vi "SV TDMS Write Spectrum (Colormap).vi"(0 "tdms file":refnum<k34>, 5 "group name in":string="Colormap", 9 "colormap":T7, 11 "error in":errorcluster, 13 "spectrum info":T1 {"x-axis units" items=["Time (s)"=0, "Frequency-CB (Hz)"=1, "Frequency-CPB (Hz)"=1248, "Frequency-Arbitrary (Hz)"=2357, "Quefrency (s)"=2, "Revolutions (rev)"=3, "Order"=4, "Speed (RPM)"=11, "Speed (rad/s)"=21, "Index"=65535]; "weighting filter" items=["Linear", "A-weighting", "B-weighting", "C-weighting", "ITU-R 468-4", "Dolby", "CCITT", "C-message", "Wb", "Wc", "Wd", "We", "Wf", "Wh", "Wj", "Wk", "Wm", "AES17 20 kHz lowpass", "AES17 40 kHz lowpass", "AES17 20 kHz highpass", "AES17 40 kHz highpass"]; "dB reference [EU]" format="%.2f"; "engineering units" items=["custom..."=0, "V"=1, "A"=21, "C"=30, "pC"=31, "s"=32, "-"=29, "Pa"=2, "N"=20, "g"=3, "m/s^2"=4, "m/s"=5, "m"=6, "mm/s"=12, "mm"=13, "micron/s"=14, "micron"=15, "in/s^2"=7, "in/s"=8, "in"=9, "mil/s"=10, "mil"=11, "rad/s^2"=16, "rad/s"=17, "rad"=18, "deg/s^2"=26, "deg/s"=27, "deg"=28, "RPM"=22, "cycle/s^2"=23, "Hz"=24, "cycle"=25, "strain"=19]; "spectral info"."window" items=["None "=0, "Hanning"=1, "Hamming"=2, "Blackman-Harris"=3, "Exact Blackman"=4, "Blackman"=5, "Flat Top"=6, "4 Term B-Harris "=7, "7 Term B-Harris"=8, "Low Sidelobe"=9, "Force - Exponential"=10, "Gaussian"=62]}) -> (4 "tdms file out":refnum<k34>, 6 "group name out":string="Colormap", 15 "error out":errorcluster)   [LabVIEW 2017]
doc: "Writes data to the specified .tdms file in a format specific to the polymorphic instance. Wire data to the <B>scaled signal [EU]</B> input to determine the polymorphic instance to use or manually select the instance."
uses:
  <vilib>/addons/_NISVFA/_Shared subVIs/Controls/svc_Spectrum Info.ctl
  <vilib>/addons/_NISVFA/_Shared subVIs/Controls/svc_X-Axis Units.ctl
  <vilib>/addons/_NISVFA/_Shared subVIs/Controls/svc_Spectrum Type.ctl
  <vilib>/addons/_NISVFA/_Shared subVIs/Controls/svc_Engineering Units Text Ring.ctl
  <vilib>/addons/_NISVFA/_Shared subVIs/Controls/svc_Weighting Filter Text Ring.ctl
  <vilib>/addons/_NISVFA/_Shared subVIs/Controls/svc_Complimentary Spectrum Units.ctl
  <vilib>/addons/_NISVFA/_Shared subVIs/Controls/svc_Speed Profile.ctl
  <vilib>/addons/_NISVFA/_Shared subVIs/Controls/NI Channel Properties.ctl
  <vilib>/addons/_NISVFA/_Shared subVIs/Controls/LV Datatypes.ctl
  <vilib>/addons/_NISVFA/_Shared subVIs/Controls/NI Spectrum Component.ctl
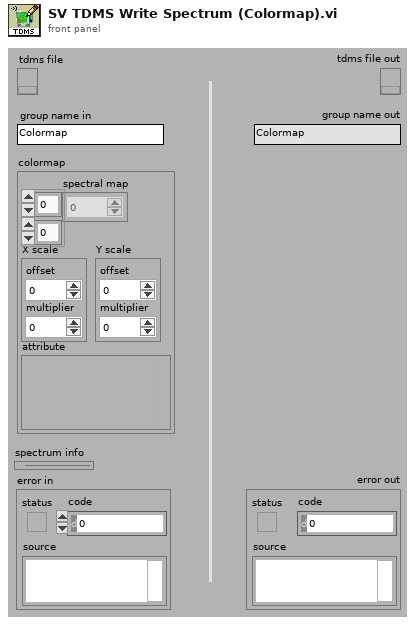
[diagram p1: front panel]
types:
  T1 = typedef "svc_Spectrum Info.ctl" = cluster{"channel name":string, "description":string, "x-axis units":T2, "spectral info":cluster{"spectrum type":T3, "linear/dB":enum16{"linear", "dB"}, "window":u16, "window size":i32, "FFT size":i32}, "engineering units":T4, "custom label":string, "dB reference [EU]":dbl, "peak units":enum16{"rms", "peak", "peak-peak"}, "weighting filter":T5, "spectral density?":bool, "unit label":string, "spectrum skewed?":bool, "complimentary spectrum units":T6}
  T2 = typedef "svc_X-Axis Units.ctl" = u16
  T3 = typedef "svc_Spectrum Type.ctl" = enum16{"FFT Spectrum [complex]", "Amplitude [Magnitude]", "Power [Magnitude^2]", "Cross Spectrum [complex]", "Frequency Response [Complex]"}
  T4 = typedef "svc_Engineering Units Text Ring.ctl" = u16
  T5 = typedef "svc_Weighting Filter Text Ring.ctl" = u16
  T6 = typedef "svc_Complimentary Spectrum Units.ctl" = enum16{"none", "radians", "degrees", "cycles", "imaginary"}
  T7 = cluster{"spectral map":dbl[][], "X scale":cluster{"offset":dbl, "multiplier":dbl}, "Y scale":cluster{"offset":dbl, "multiplier":dbl}, "attribute":variant}
  T8 = typedef "LV Datatypes.ctl" = i32
  T9 = typedef "NI Spectrum Component.ctl" = u16
  T10 = typedef "NI Channel Properties.ctl" = u16
  T11 = enum16{"Frequency-Time", "Time-Frequency", "Order-Time", "Time-Order", "Frequency-RPM", "RPM-Frequency", "Order-RPM", "RPM-Order"}
  T12 = typedef "svc_Speed Profile.ctl" = cluster{"time [s]":dbl[], "speed [RPM]":dbl[]}
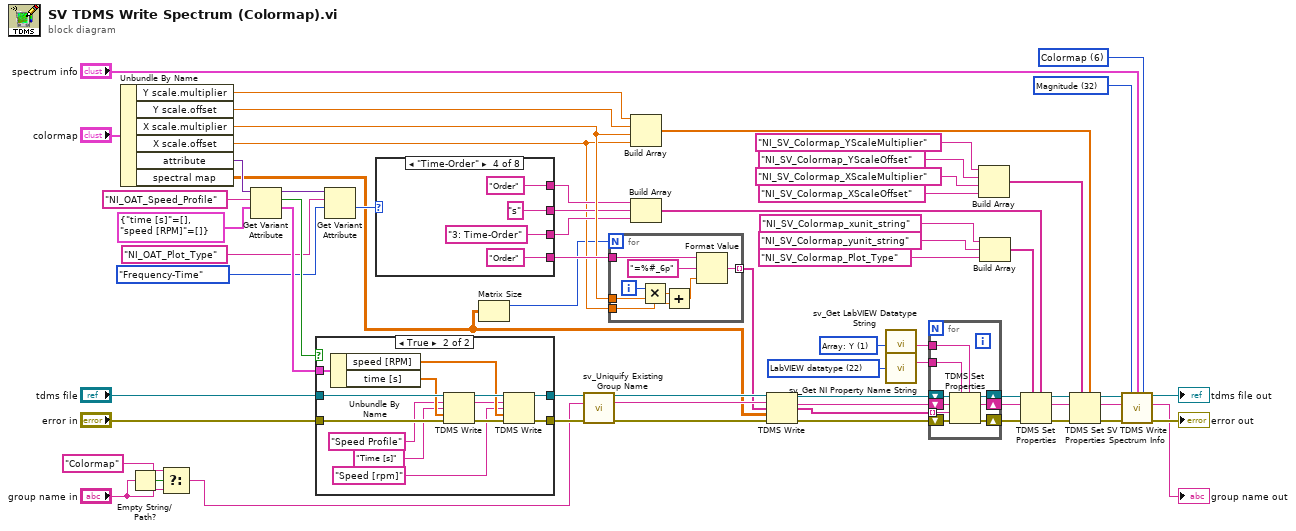
[diagram p0: block diagram]
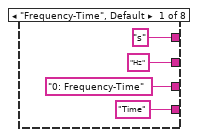
[diagram p2: hidden frame]
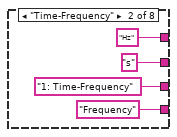
[diagram p3: hidden frame]
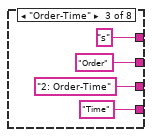
[diagram p4: hidden frame]
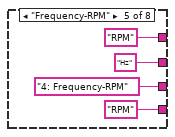
[diagram p5: hidden frame]
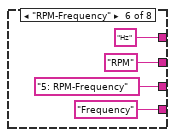
[diagram p6: hidden frame]
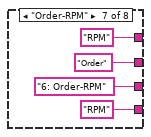
[diagram p7: hidden frame]
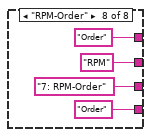
[diagram p8: hidden frame]
diagram:
  w35 = T8 6 items=["String: abc"=7, "Boolean: True or False"=8, "Scalar: y"=0, "Array: Y"=1, "Waveform: t0, dt, Y, variant"=2, "Cluster: x0, dx, Y"=3, "Cluster: X, Y"=4, "Waterfall"=5, "Colormap"=6] ("LabVIEW datatype")
  w41 = T9 32 items=["Magnitude"=32, "Phase"=33, "Real"=34, "Imaginary"=35, "Coherence"=36, "Unknown"=99] ("spectrum component")
  w52 = T8 1 items=["String: abc"=-2, "Boolean: True or False"=-1, "Scalar: y"=0, "Array: Y"=1, "Waveform: t0, dt, Y, variant"=2, "Cluster: x0, dx, Y"=3, "Cluster: X, Y"=4, "Waterfall"=5, "Colormap"=6] ("LabVIEW datatype")
  w53 = T10 22 items=["Channel name", "Channel description", "Y-axis label", "Y-axis unit string", "X-axis label", "X-axis unit string", "x0", "dx", "Number of samples", "X channel", "Filter settled", "dB reference", "Window", "Window parameter", "Window size", "FFT size", "Peak units", "Spectrum type", "Magnitude scale", "Spectral density", "Sensor sensitivity (mV/EU)", "X-axis domain", "LabVIEW datatype"] ("property")
  n1 = Unbundle By Name("colormap") -> ("Y scale.multiplier"=w28:dbl, "Y scale.offset"=w27:dbl, "X scale.multiplier"=w26:dbl, "X scale.offset"=w4:dbl, "attribute"=w60:variant, "spectral map"=w2:dbl[][])
  n2 = Empty String/Path?(string/path="group name in") -> (empty?=w64:bool)
  n3 = Select(t="Colormap" ("group name"), s=w64, f="group name in") -> (s? t:f=w3:string)
  n4 = Get Variant Attribute(Variant=w60, name="NI_OAT_Speed_Profile", default value (empty Variant)=T12 {"time [s]"=[], "speed [RPM]"=[]} ("speed profile")) -> (duplicate Variant=w61:variant, found=w59:bool, value=w58:T12)  [unwired: 1 in, 1 out]
  n5 = case shown="True" w59 {
    tunnel: "tdms file" -> [w68 w81]
    tunnel: "error in" -> [w67 w80]
    tunnel: [w67 w77] -> w38
    tunnel: [w68 w76] -> w40
    tunnel: w58 -> [_ w75]
    frame False {
    }
    frame True {
      n6 = Unbundle By Name(w75) -> ("speed [RPM]"=w73:dbl[], "time [s]"=w74:dbl[])
      n7 = TDMS Write(0:w81, 5:"Speed Profile" ("name"), 7:"Time [s]" ("name"), 9:w74, 11:w80) -> (4:w79:refnum<k34>, 6:w69:string, 15:w78:errorcluster)  [unwired: 1 in, 1 out]
      n8 = TDMS Write(0:w79, 5:w69, 7:"Speed [rpm]" ("name"), 9:w73, 11:w78) -> (4:w76:refnum<k34>, 15:w77:errorcluster)  [unwired: 1 in, 2 out]
    }
  }
  n9 = Get Variant Attribute(Variant=w61, name="NI_OAT_Plot_Type", default value (empty Variant)=T11."Frequency-Time" ("plot type")) -> (value=w31:T11)  [unwired: 1 in, 3 out]
  n10 = case shown="\"Time-Order\"" w31 {
    tunnel: ["s" ("name") "Hz" ("name") "s" ("name") "Order" ("name") "RPM" ("name") "Hz" ("name") "RPM" ("name") "Order" ("name")] -> w16
    tunnel: ["Hz" ("name") "s" ("name") "Order" ("name") "s" ("name") "Hz" ("name") "RPM" ("name") "Order" ("name") "RPM" ("name")] -> w15
    tunnel: ["0: Frequency-Time" "1: Time-Frequency" "2: Order-Time" "3: Time-Order" "4: Frequency-RPM" "5: RPM-Frequency" "6: Order-RPM" "7: RPM-Order"] -> w14
    tunnel: ["Time" ("name") "Frequency" ("name") "Time" ("name") "Order" ("name") "RPM" ("name") "Frequency" ("name") "RPM" ("name") "Order" ("name")] -> w30
    frame "Frequency-Time", Default {
    }
    frame "Time-Frequency" {
    }
    frame "Order-Time" {
    }
    frame "Time-Order" {
    }
    frame "Frequency-RPM" {
    }
    frame "RPM-Frequency" {
    }
    frame "Order-RPM" {
    }
    frame "RPM-Order" {
    }
  }
  n11 = Matrix Size(0:w2) -> (1:w1:i32)  [unwired: 1 out]
  n12 = call <vilib>:"sv_Uniquify Existing Group Name.vi"("tdms file ref"=w40, "group name"=w3, "error in"=w38) -> ("tdms file out"=w39:refnum<k34>, "unique group"=w36:string, "error out"=w37:errorcluster)  [unwired: 10 in]
  n13 = for {
    N: w1 -> [_]
    tunnel: [w121] -> w5 mode=indexing
    tunnel: w26 -> [w120]
    tunnel: w4 -> [w119]
    tunnel: w30 -> [w117]
    i -> [w118]
    n14 = Multiply(x=w118, y=w120) -> (x*y=w116:dbl)
    n15 = Add(x=w116, y=w119) -> (x+y=w115:dbl)
    n16 = Format Value(string ("")=w117, format string="=%#_6p", value (0)=w115) -> (output string=w121:string)
  }
  n17 = Build Array(w28, w27, w26, w4) -> (w17:dbl[])
  n18 = Build Array(w16, w15, w14) -> (w9:string[])
  n19 = TDMS Write(0:w39, 5:w36, 7:w5, 9:w2, 11:w37) -> (4:w49:refnum<k34>, 6:w50:string, 8:w48:string[], 15:w51:errorcluster)  [unwired: 1 in]
  n20 = call <vilib>:"sv_Get LabVIEW Datatype String.vi"("LabVIEW datatype"=w52) -> ("datatype string"=w47:string)  [unwired: 4 in]
  n21 = call <vilib>:"sv_Get NI Property Name String.vi"("property"=w53) -> ("TDMS property name"=w46:string)  [unwired: 13 in, 1 out]
  n22 = for {
    tunnel: w48 -> [w127] mode=indexing
    tunnel: w47 -> [w126]
    tunnel: w46 -> [w125]
    shift-right: [w124] -> w45
    shift-left: w49 -> [w128]
    shift-right: [w123] -> w44
    shift-left: w50 -> [w129]
    shift-right: [w122] -> w43
    shift-left: w51 -> [w130]
    n23 = TDMS Set Properties(5:w126, 7:w125, 8:w130, 9:w127, 10:w129, 11:w128) -> (0:w122:errorcluster, 2:w123:string, 3:w124:refnum<k34>)  [unwired: 1 out]
  }
  n24 = Build Array("NI_SV_Colormap_YScaleMultiplier" ("channel name"), "NI_SV_Colormap_YScaleOffset" ("channel name"), "NI_SV_Colormap_XScaleMultiplier" ("channel name"), "NI_SV_Colormap_XScaleOffset" ("channel name")) -> (w21:string[])
  n25 = Build Array("NI_SV_Colormap_xunit_string" ("channel name"), "NI_SV_Colormap_yunit_string" ("channel name"), "NI_SV_Colormap_Plot_Type" ("name")) -> (w10:string[])
  n26 = TDMS Set Properties(5:w9, 7:w10, 8:w43, 10:w44, 11:w45) -> (0:w18:errorcluster, 2:w19:string, 3:w20:refnum<k34>)  [unwired: 1 in, 1 out]
  n27 = TDMS Set Properties(5:w17, 7:w21, 8:w18, 10:w19, 11:w20) -> (0:w8:errorcluster, 2:w7:string, 3:w6:refnum<k34>)  [unwired: 1 in, 1 out]
  n28 = call <vilib>:"SV TDMS Write Spectrum Info.vi"("tdms file"=w6, "spectrum component"=w41, "spectrum info"="spectrum info", "LabVIEW datatype"=w35, "group name in"=w7, "error in"=w8) -> ("tdms file out"=→"tdms file out":refnum<k34>, "group name out"=→"group name out":string, "error out"=→"error out":errorcluster)  [unwired: 4 in, 3 out]
